vi "ge_FindChassis.vi"(8 "error in":errorcluster) -> (0 "error out":errorcluster, 1 "Meta data":T1[](array[typedef]), 3 "cDAQ Configs":T2[](array[typedef]))   [LabVIEW 2012]
uses:
  Custom Ctrls/Master Cfg/ge_Cfg wChassis.ctl
  Classes/Cfg Grandmaster/Class Chassis Cfg/ChassisCfg.lvclass
  Classes/Cfg Grandmaster/Class Chassis BOM/Chassis BOM.lvclass
  <userlib>/STM/_SubVIs/stm_MetaDataElement.ctl
  Custom Ctrls/ge_AMC_Qname.ctl
  Custom Ctrls/ge_ChassisType.ctl
  <resource>/objmgr/daqmx.rc
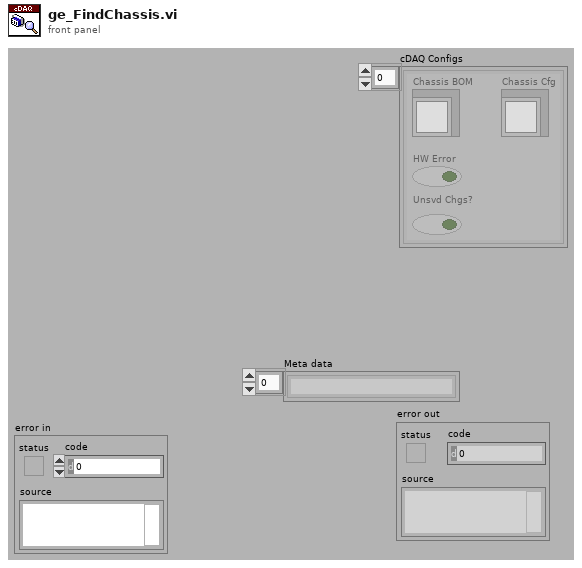
[diagram p1: front panel]
types:
  T1 = typedef "stm_MetaDataElement.ctl" = string
  T2 = typedef "ge_Cfg wChassis.ctl" = cluster{"Chassis BOM":refnum<class "Chassis BOM.lvclass">, "Chassis Cfg":refnum<class "ChassisCfg.lvclass">, "HW Error":bool, "Unsvd Chgs?":bool}
  T3 = typedef "ge_AMC_Qname.ctl" = enum16{"Cmnd Loop", "UI Updater", "Conn Mgr HS", "Conn Mgr LS", "TCP Send HS", "TCP Send LS"}
  T4 = typedef "ge_ChassisType.ctl" = enum16{"Not Supported", "1-Slot", "4-Slot", "8-Slot"}
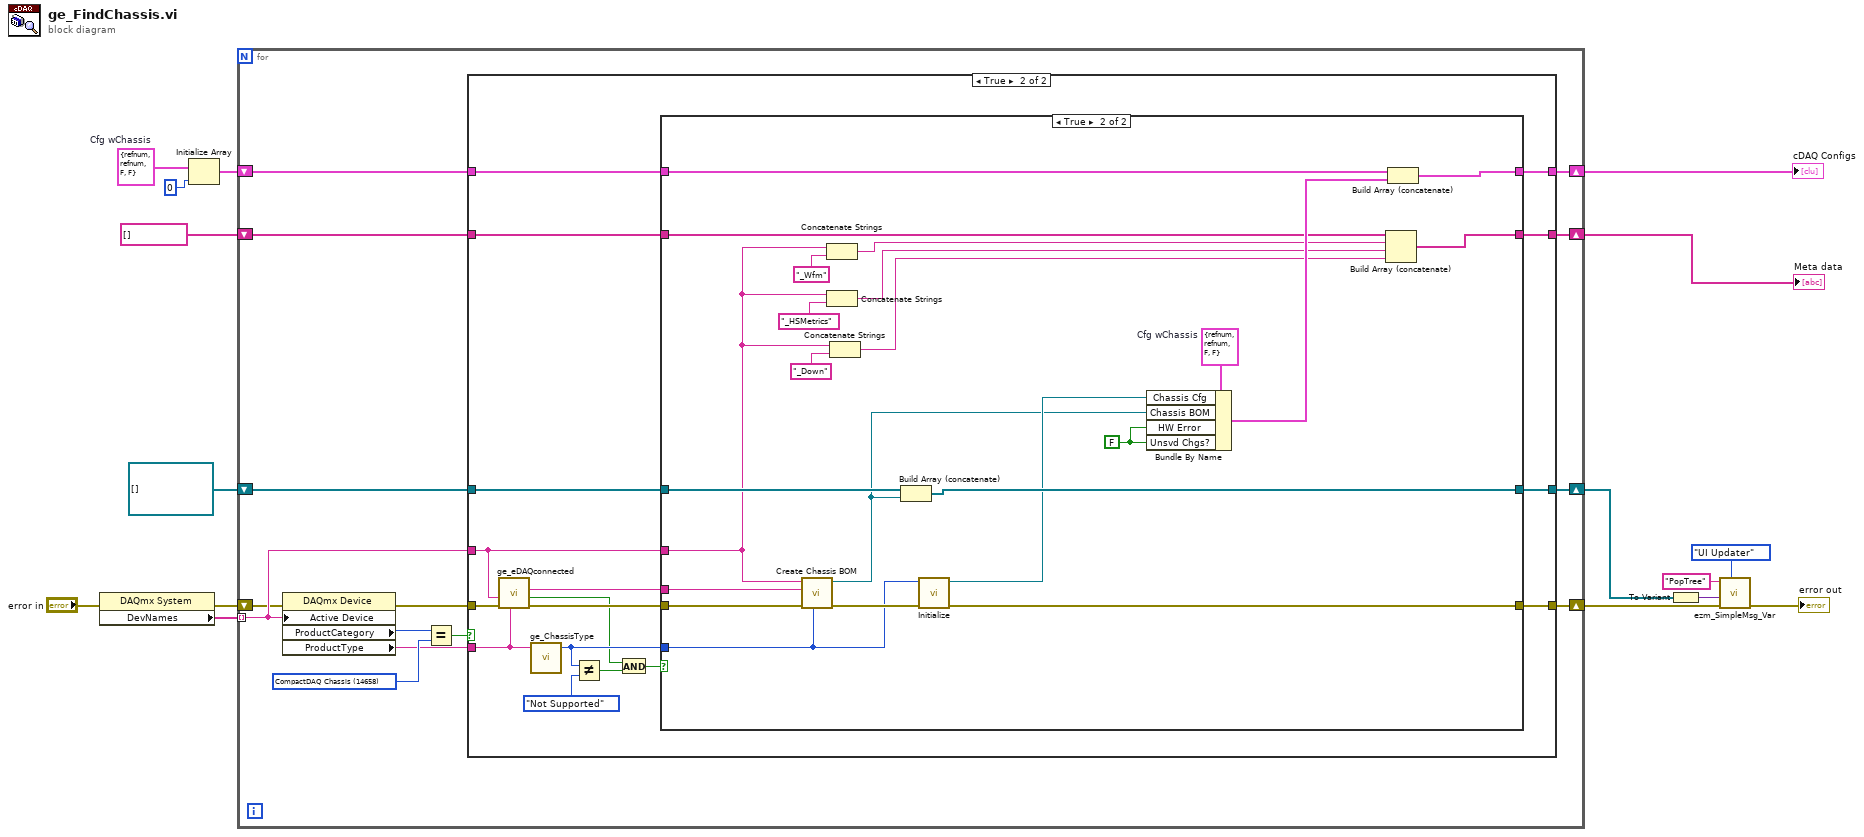
[diagram p0: block diagram]
diagram:
  w6 = T2 {"Chassis BOM"=refnum, "Chassis Cfg"=refnum, "HW Error"=FALSE, "Unsvd Chgs?"=FALSE}  # Cfg wChassis
  n1 = property class="DAQmx System"(error in="error in") -> (error out=w14:errorcluster, "DevNames"=w15:tag[])  [unwired: 1 in, 1 out]
  n2 = Initialize Array(w6, 0 ("dimension size")) -> (w8:T2[])
  n3 = for {
    tunnel: w15 -> [w28] mode=indexing
    shift-right: [w25] -> w12
    shift-left: w14 -> [w27]
    shift-right: [w23] -> w7
    shift-left: w8 -> [w24]
    shift-right: [w21] -> w10
    shift-left: refnum<class "Chassis BOM.lvclass">[] [] -> [w22]
    shift-right: [w19] -> w4
    shift-left: T1[] [] ("Meta data") -> [w20]
    w30 = 14658 items=["M Series DAQ"=14643, "X Series DAQ"=15858, "E Series DAQ"=14642, "S Series DAQ"=14644, "B Series DAQ"=14662, "SC Series DAQ"=14645, "USB DAQ"=14646, "AO Series"=14647, "Digital I/O"=14648, "TIO Series"=14661, "Dynamic Signal Acquisition"=14649, "Switches"=14650, "CompactDAQ Chassis"=14658, "C Series Module"=14659, "SCXI Module"=14660, "SCC Connector Block"=14704, "SCC Module"=14705, "NI ELVIS"=14755, "Network DAQ"=14829, "SC Express"=15886, "Unknown"=12588] ("ProductCategory")
    n4 = property class="DAQmx Device"(error in=w27, "Active Device"=w28) -> (error out=w26:errorcluster, "ProductCategory"=w18:i32, "ProductType"=w17:string)  [unwired: 1 in, 1 out]
    n5 = Equal?(x=w18, y=w30) -> (x = y?=w29:bool)
    n6 = case shown="True" w29 {
      tunnel: w28 -> [_ w44]
      tunnel: w26 -> [w34 w46]
      tunnel: [w34 w47] -> w25
      tunnel: w24 -> [w33 w51]
      tunnel: [w33 w50] -> w23
      tunnel: w22 -> [w32 w49]
      tunnel: [w32 w48] -> w21
      tunnel: w20 -> [w31 w43]
      tunnel: [w31 w42] -> w19
      tunnel: w17 -> [_ w36]
      frame False {
      }
      frame True {
        n7 = call "ge_eDAQconnected.vi"("ProductType"=w36, "error in"=w46, "DAQmx Device Name"=w44) -> ("error out"=w45:errorcluster, "Device Connected?"=w39:bool, "TCPIP.EthernetIP"=w35:string)  [unwired: 6 in]
        n8 = call "ge_ChassisType.vi"("ProductType"=w36) -> ("ChassisType"=w41:T4)  [unwired: 4 in]
        n9 = Not Equal?(x=w41, y=ge_ChassisType."Not Supported") -> (x != y?=w38:bool)
        n10 = And(x=w39, y=w38) -> (x .and. y?=w37:bool)
        n11 = case shown="True" w37 {
          tunnel: w51 -> [w53 w78]
          tunnel: [w53 w77] -> w50
          tunnel: w49 -> [w54 w76]
          tunnel: [w54 w75] -> w48
          tunnel: [w55 w62] -> w47
          tunnel: w44 -> [_ w60]
          tunnel: w45 -> [w55 w59]
          tunnel: w43 -> [w52 w71]
          tunnel: [w52 w70] -> w42
          tunnel: w41 -> [_ w57]
          tunnel: w35 -> [_ w61]
          frame False {
          }
          frame True {
            w72 = FALSE ("HW Error")
            w74 = T2 {"Chassis BOM"=refnum, "Chassis Cfg"=refnum, "HW Error"=FALSE, "Unsvd Chgs?"=FALSE}  # Cfg wChassis
            n12 = call "Create Chassis BOM.vi"("ChassisType"=w57, "error in (no error)"=w59, "TCPIP.EthernetIP"=w61, "DAQmx Device Name"=w60) -> ("error out"=w58:errorcluster, "Chassis BOM out"=w56:refnum<class "Chassis BOM.lvclass">)  [unwired: 6 in]
            n13 = Concatenate Strings(w60, "_Wfm") -> (w68:string)
            n14 = Concatenate Strings(w60, "_HSMetrics") -> (w66:string)
            n15 = Concatenate Strings(w60, "_Down") -> (w64:string)
            n16 = Build Array (concatenate)(w76, w56) -> (w75:refnum<class "Chassis BOM.lvclass">[])
            n17 = call "Initialize.vi"("error in"=w58, "ChassisType"=w57) -> ("error out"=w62:errorcluster, "Chassis Cfg"=w63:refnum<class "ChassisCfg.lvclass">)  [unwired: 7 in]
            n18 = Bundle By Name(cluster=w74, "Chassis Cfg"=w63, "Chassis BOM"=w56, "HW Error"=w72, "Unsvd Chgs?"=w72) -> (w73:T2)
            n19 = Build Array (concatenate)(w71, w68, w66, w64) -> (w70:T1[])
            n20 = Build Array (concatenate)(w78, w73) -> (w77:T2[])
          }
        }
      }
    }
  }
  "cDAQ Configs" <- w7
  "Meta data" <- w4
  n21 = To Variant(anything=w10) -> (Variant=w2:variant)
  n22 = call "ezm_SimpleMsg_Var.vi"("Destination Queue"=ge_AMC_Qname."UI Updater" ("ge_AMC_Qname"), "error in"=w12, "Msg Data"=w2, "Msg Name"="PopTree") -> ("error out"=→"error out":errorcluster)  [unwired: 6 in, 1 out]
